vi "LoadImageFromString.vi"(1 "ImageFileContent":string, 3 "ImageFileFileExtention(png,jpg,...)":string, 5 "error in (no error)":errorcluster) -> (15 "ImageOut":refnum<k24>, 17 "ImageSize":cluster{"Width":i32, "Height":i32}, 19 "error out":errorcluster)   [LabVIEW 2019, in "LcPictureBox.lvclass"]
uses:
  LcPictureBox.lvclass
  System.Drawing
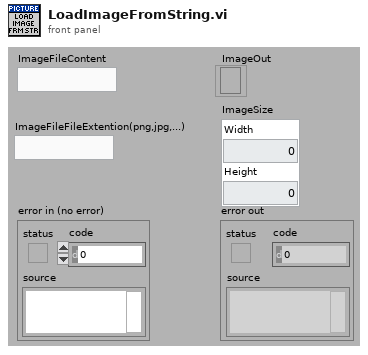
[diagram p1: front panel]
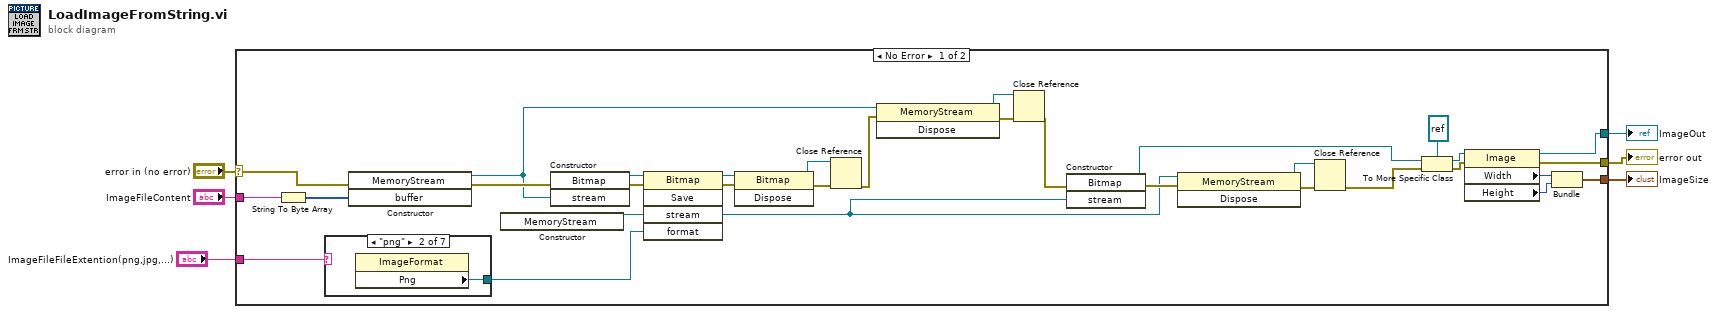
[diagram p0: block diagram]
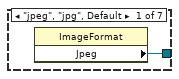
[diagram p2: hidden frame]
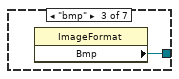
[diagram p3: hidden frame]
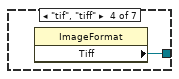
[diagram p4: hidden frame]
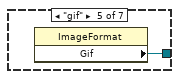
[diagram p5: hidden frame]
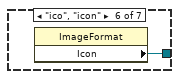
[diagram p6: hidden frame]
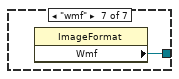
[diagram p7: hidden frame]
diagram:
  n1 = case shown="No Error" "error in (no error)" {
    selector: "error in (no error)" -> [w14 w45]
    tunnel: [w33 w45] -> w5
    tunnel: "ImageFileContent" -> [w15 _]
    tunnel: [w35 _] -> w4
    tunnel: [w30 _] -> w3
    tunnel: "ImageFileFileExtention(png,jpg,...)" -> [w12 _]
    frame No Error {
      n2 = String To Byte Array(string=w15) -> (unsigned byte array=w16:u8[])
      n3 = case shown="\"png\"" w12 {
        tunnel: [w38 w39 w40 w41 w42 w43 w44] -> w27
        frame "jpeg", "jpg", Default {
          n4 = property class="ImageFormat"() -> ("Jpeg"=w38:refnum<k24>)  [unwired: 2 in, 2 out]
        }
        frame "png" {
          n5 = property class="ImageFormat"() -> ("Png"=w39:refnum<k24>)  [unwired: 2 in, 2 out]
        }
        frame "bmp" {
          n6 = property class="ImageFormat"() -> ("Bmp"=w40:refnum<k24>)  [unwired: 2 in, 2 out]
        }
        frame "tif", "tiff" {
          n7 = property class="ImageFormat"() -> ("Tiff"=w41:refnum<k24>)  [unwired: 2 in, 2 out]
        }
        frame "gif" {
          n8 = property class="ImageFormat"() -> ("Gif"=w42:refnum<k24>)  [unwired: 2 in, 2 out]
        }
        frame "ico", "icon" {
          n9 = property class="ImageFormat"() -> ("Icon"=w43:refnum<k24>)  [unwired: 2 in, 2 out]
        }
        frame "wmf" {
          n10 = property class="ImageFormat"() -> ("Wmf"=w44:refnum<k24>)  [unwired: 2 in, 2 out]
        }
      }
      n11 = constructor class="MemoryStream"(error in=w14, "buffer"=w16) -> (reference out=w9:refnum<k24>, error out=w13:errorcluster)  [unwired: 2 in, 2 out]
      n12 = constructor class="MemoryStream"() -> (reference out=w21:refnum<k24>)  [unwired: 3 in, 2 out]
      n13 = constructor class="Bitmap"(error in=w13, "stream"=w9) -> (reference out=w29:refnum<k24>, error out=w28:errorcluster)  [unwired: 2 in, 2 out]
      n14 = invoke class="Bitmap" method="Save"(reference=w29, error in=w28, "stream"=w21, "format"=w27) -> (reference out=w25:refnum<k24>, error out=w26:errorcluster)  [unwired: 1 in, 3 out]
      n15 = invoke class="Bitmap" method="Dispose"(reference=w25, error in=w26) -> (reference out=w23:refnum<k24>, error out=w24:errorcluster)  [unwired: 1 in, 1 out]
      n16 = Close Reference(reference=w23, error in (no error)=w24) -> (error out=w8:errorcluster)
      n17 = invoke class="MemoryStream" method="Dispose"(reference=w9, error in=w8) -> (reference out=w11:refnum<k24>, error out=w10:errorcluster)  [unwired: 1 in, 1 out]
      n18 = Close Reference(reference=w11, error in (no error)=w10) -> (error out=w7:errorcluster)
      n19 = constructor class="Bitmap"(error in=w7, "stream"=w21) -> (reference out=w17:refnum<k24>, error out=w22:errorcluster)  [unwired: 2 in, 2 out]
      n20 = invoke class="MemoryStream" method="Dispose"(reference=w21, error in=w22) -> (reference out=w19:refnum<k24>, error out=w20:errorcluster)  [unwired: 1 in, 1 out]
      n21 = Close Reference(reference=w19, error in (no error)=w20) -> (error out=w18:errorcluster)
      n22 = To More Specific Class(target class=refnum<k24> refnum, reference=w17, error in=w18) -> (specific class reference=w36:refnum<k24>, error out=w34:errorcluster)
      n23 = property class="Image"(reference=w36, error in=w34) -> (reference out=w35:refnum<k24>, error out=w33:errorcluster, "Width"=w32:i32, "Height"=w31:i32)
      n24 = Bundle("Width"=w32, "Height"=w31) -> (w30:cluster{"Width":i32, "Height":i32})  [unwired: 1 in]
    }
    frame Error {
    }
  }
  "error out" <- w5
  "ImageOut" <- w4
  "ImageSize" <- w3
